vi "Untitled 1.vi"() -> ()   [LabVIEW 2017]
panel:
  out "WDWArray 2.4":T1
  out "WDWArray 2.3":T1
  out "WDWArray 2.2":T1
  out "WDWArray 2.1":T1
  out "WDWArray 1.4":T1
  out "WDWArray 1.3":T1
  out "WDWArray 1.2":T1
  out "WDWArray 1.1":T1
  out "WDW_2_OK":bool
  out "WDW_1_OK":bool
  out "ST_WDW_Read 2":bool
  out "ST_WDW_Read 1":bool
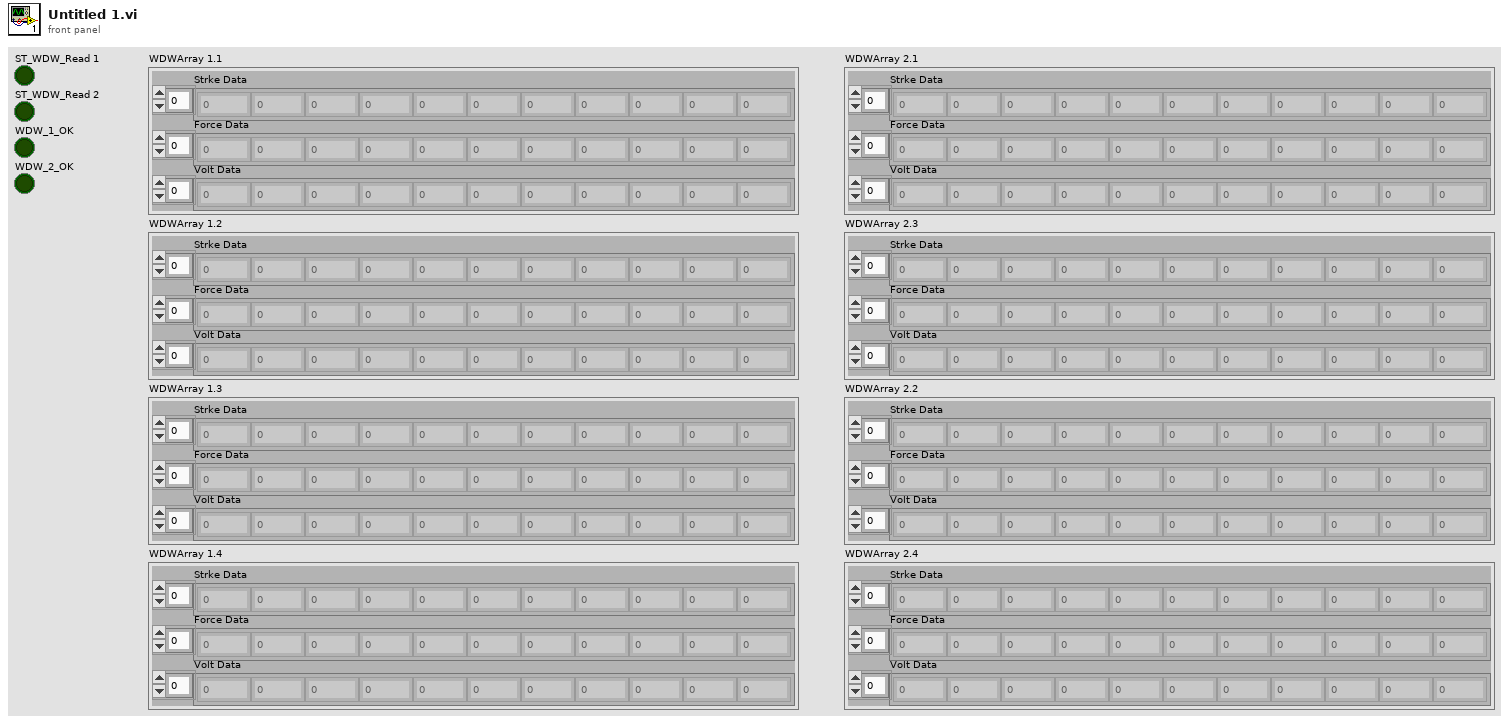
[diagram p1: front panel]
types:
  T1 = cluster{"Strke Data":dbl[], "Force Data":dbl[], "Volt Data":dbl[]}
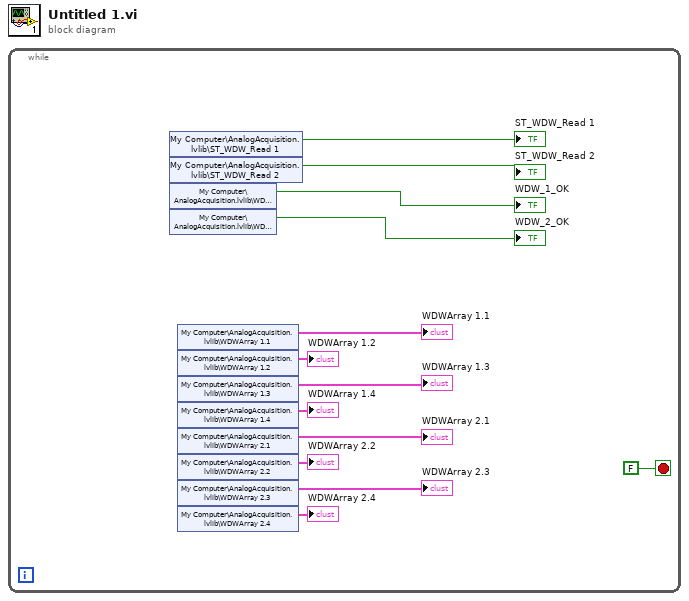
[diagram p0: block diagram]
diagram:
  n1 = while {
    stop <- FALSE stop-if-true
    n2 = shared-variable "My Computer\\AnalogAcquisition.lvlib\\ST_WDW_Read 1"() -> (→"ST_WDW_Read 1":bool)  [unwired: 1 in, 1 out]
    n3 = shared-variable "My Computer\\AnalogAcquisition.lvlib\\ST_WDW_Read 2"() -> (→"ST_WDW_Read 2":bool)  [unwired: 1 in, 1 out]
    n4 = shared-variable "My Computer\\AnalogAcquisition.lvlib\\WDW_1_OK"() -> (→"WDW_1_OK":bool)  [unwired: 1 in, 1 out]
    n5 = shared-variable "My Computer\\AnalogAcquisition.lvlib\\WDW_2_OK"() -> (→"WDW_2_OK":bool)  [unwired: 1 in, 1 out]
    n6 = shared-variable "My Computer\\AnalogAcquisition.lvlib\\WDWArray 1.1"() -> (→"WDWArray 1.1":T1)  [unwired: 1 in, 1 out]
    n7 = shared-variable "My Computer\\AnalogAcquisition.lvlib\\WDWArray 1.2"() -> (→"WDWArray 1.2":T1)  [unwired: 1 in, 1 out]
    n8 = shared-variable "My Computer\\AnalogAcquisition.lvlib\\WDWArray 1.3"() -> (→"WDWArray 1.3":T1)  [unwired: 1 in, 1 out]
    n9 = shared-variable "My Computer\\AnalogAcquisition.lvlib\\WDWArray 1.4"() -> (→"WDWArray 1.4":T1)  [unwired: 1 in, 1 out]
    n10 = shared-variable "My Computer\\AnalogAcquisition.lvlib\\WDWArray 2.1"() -> (→"WDWArray 2.1":T1)  [unwired: 1 in, 1 out]
    n11 = shared-variable "My Computer\\AnalogAcquisition.lvlib\\WDWArray 2.2"() -> (→"WDWArray 2.2":T1)  [unwired: 1 in, 1 out]
    n12 = shared-variable "My Computer\\AnalogAcquisition.lvlib\\WDWArray 2.3"() -> (→"WDWArray 2.3":T1)  [unwired: 1 in, 1 out]
    n13 = shared-variable "My Computer\\AnalogAcquisition.lvlib\\WDWArray 2.4"() -> (→"WDWArray 2.4":T1)  [unwired: 1 in, 1 out]
  }
